vi "uniqueLine.vi"(11 "RobotRef in":refnum<class "Robot.lvclass">[](array[class])) -> (3 "Array":refnum<class "Robot.lvclass">[](array[class]))   [LabVIEW 2020, in "Game.lvclass"]
uses:
  Game.lvclass
  Robot_class/Robot.lvclass
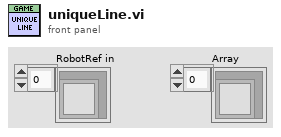
[diagram p1: front panel]
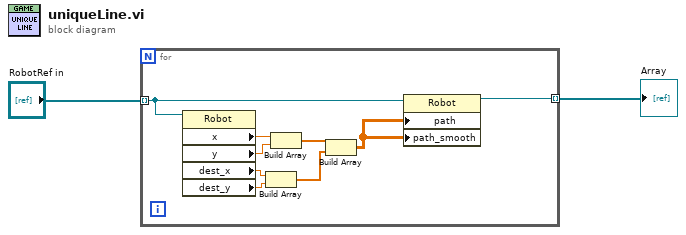
[diagram p0: block diagram]
diagram:
  n1 = for {
    tunnel: "RobotRef in" -> [w10] mode=indexing
    tunnel: [w11] -> w2 mode=indexing
    n2 = property class="Robot"(reference=w10) -> ("x"=w9:dbl, "y"=w8:dbl, "dest_x"=w7:dbl, "dest_y"=w6:dbl)  [unwired: 1 in, 2 out]
    n3 = Build Array(w7, w6) -> (w4:dbl[])
    n4 = Build Array(w9, w8) -> (w5:dbl[])
    n5 = Build Array(w5, w4) -> (w3:dbl[][])
    n6 = property class="Robot"(reference=w10, "path"=w3, "path_smooth"=w3) -> (reference out=w11:refnum<class "Robot.lvclass">)  [unwired: 1 in, 1 out]
  }
  "Array" <- w2
